vi "Process.vi"(2 "gen":refnum<class "niUSRP Tx DSP v2 FPGA.lvclass">) -> ()   [LabVIEW 2025, in "niUSRP Tx DSP v2 FPGA.lvclass"]
uses:
  niUSRP Tx DSP v2 FPGA.lvclass
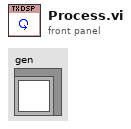
[diagram p1: front panel]
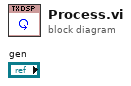
[diagram p0: block diagram]
diagram:
